vi "MAIN_check_XY_stage_positions.vi"(5 "Update display properties?":bool, 6 "error in":errorcluster, 7 "XY positions":refnum<vi>, 8 "ROI manager":i32(listbox), 9 "XY positions":dbl[][](array[numeric])) -> (0 "error out":errorcluster, 2 "XYZ":cluster{"x(um)":dbl, "y(um)":dbl, "z(um)":dbl} {"x(um)" format="%#.1f"; "y(um)" format="%#.1f"; "z(um)" format="%#.1f"}, 3 "XY positions OUT":dbl[][](array[numeric]), 4 "XY graph":cluster{dbl[], dbl[]}[](array[cluster]))   [LabVIEW 2015]
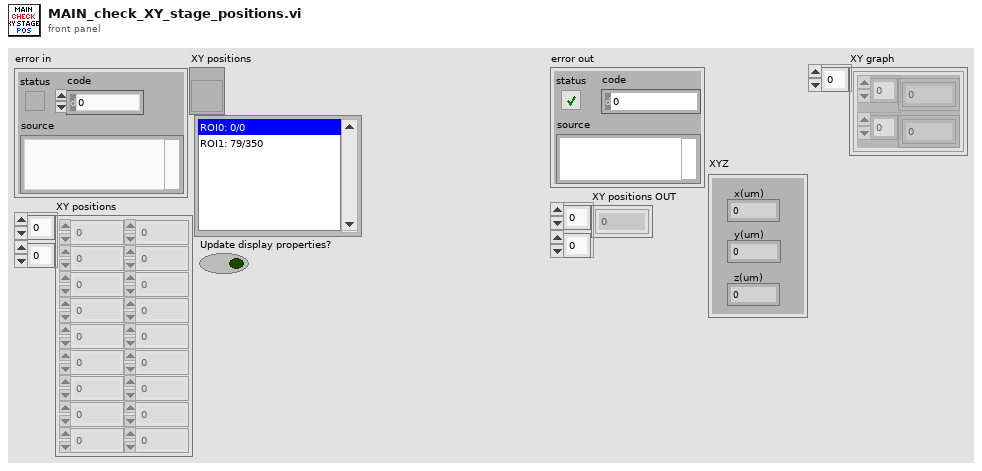
[diagram p1: front panel]
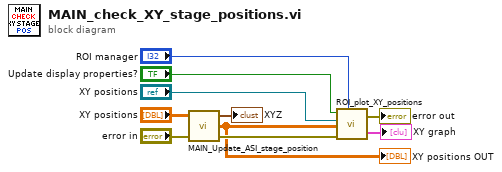
[diagram p0: block diagram]
diagram:
  n1 = call "MAIN_Update_ASI_stage_position.vi"("error in"="error in", "XY positions"="XY positions") -> ("error out"=w8:errorcluster, "XY positions OUT"=w7:dbl[][], "XYZ"=→"XYZ":cluster{"x(um)":dbl, "y(um)":dbl, "z(um)":dbl})  [unwired: 1 in]
  "XY positions OUT" <- w7
  n2 = call "ROI_plot_XY_positions.vi"("Display?"="Update display properties?", "XYGraph Refnum"="XY positions", "XY positions"=w7, "error in"=w8, "ROI manager"="ROI manager") -> ("error out"=→"error out":errorcluster, "XY graph"=→"XY graph":cluster{dbl[], dbl[]}[])
